vi "Fm.vi"() -> ()   [LabVIEW 2016]
uses:
  <vilib>/measure/NI_MAPro.lvlib
panel:
  out "Waveform Graph":dynamicdata(graph)
  in  "Kf":dbl(slide) scale=0.0..100.0
  in  "Fc":dbl(knob) scale=0.0..100.0
  in  "Ac":dbl(knob) scale=0.0..1.0
  in  "Am":dbl(knob) scale=0.0..1.0
  in  "Fm":dbl(knob) scale=0.0..10.0
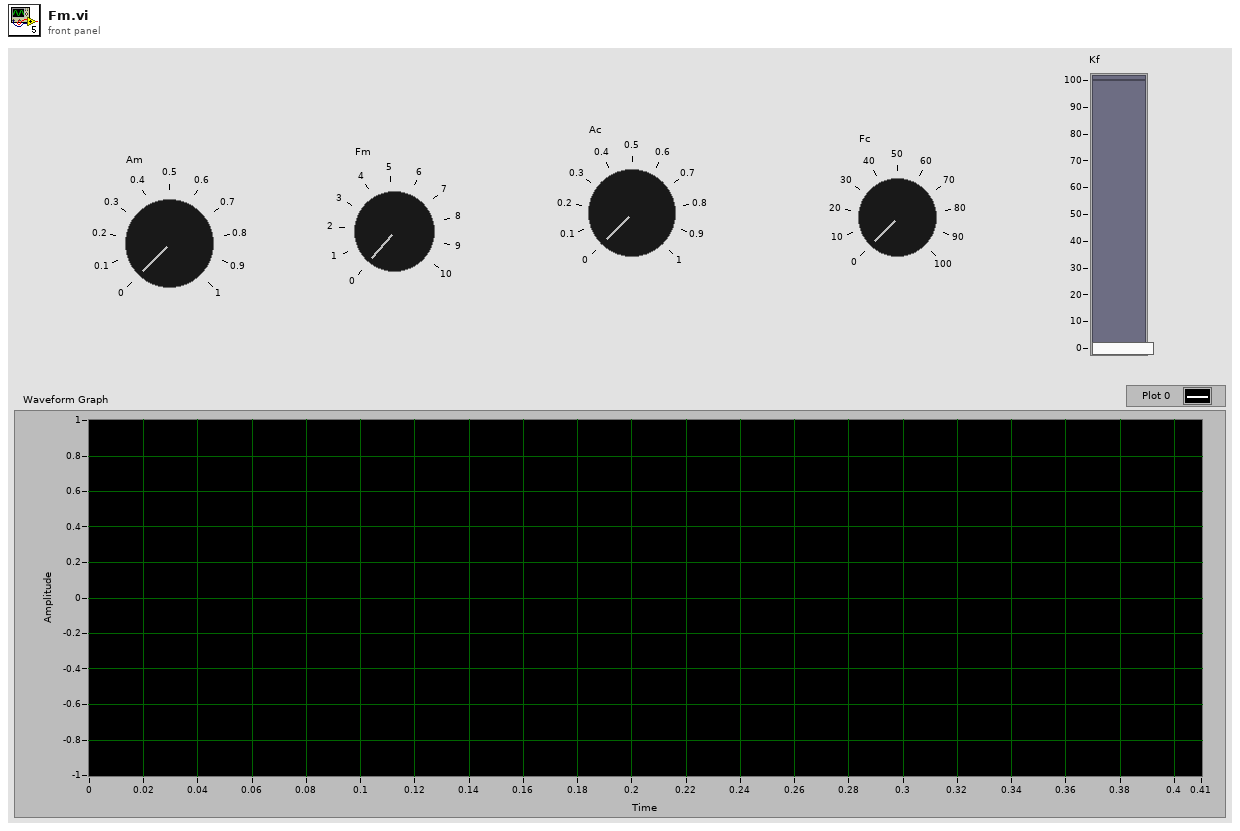
[diagram p1: front panel]
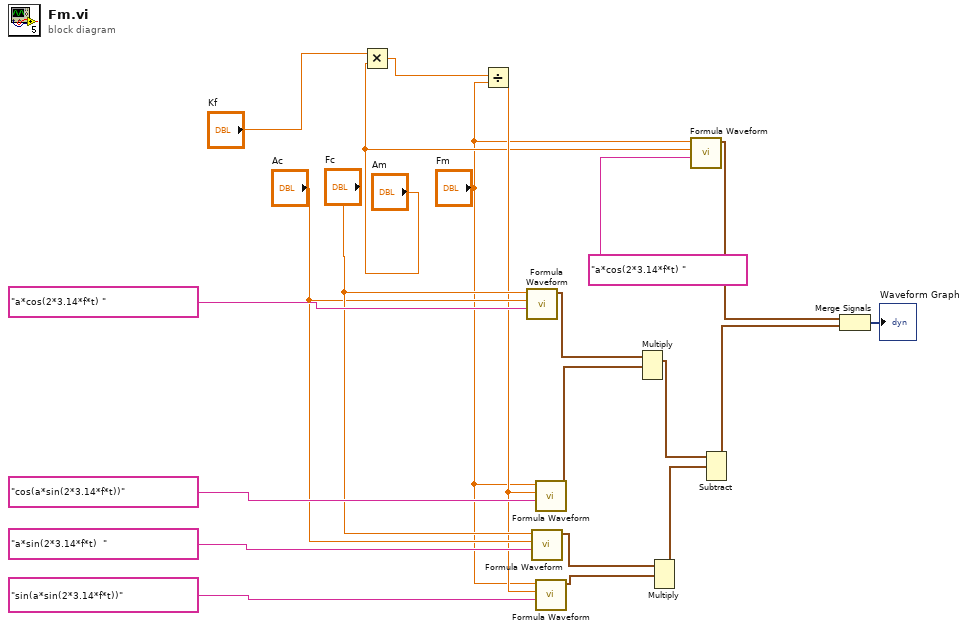
[diagram p0: block diagram]
diagram:
  n1 = Multiply(x="Kf", y="Am") -> (x*y=w14:dbl)
  n2 = Divide(x=w14, y="Fm") -> (x/y=w13:dbl)
  n3 = call <vilib>:"Formula Waveform.vi"("formula"="a*cos(2*3.14*f*t) ", "amplitude"="Ac", "frequency"="Fc") -> ("signal out"=w12:waveform(dbl))  [unwired: 7 in, 1 out]
  n4 = call <vilib>:"Formula Waveform.vi"("formula"="a*sin(2*3.14*f*t)  ", "amplitude"="Ac", "frequency"="Fc") -> ("signal out"=w10:waveform(dbl))  [unwired: 7 in, 1 out]
  n5 = call <vilib>:"Formula Waveform.vi"("formula"="cos(a*sin(2*3.14*f*t))", "amplitude"=w13, "frequency"="Fm") -> ("signal out"=w11:waveform(dbl))  [unwired: 7 in, 1 out]
  n6 = call <vilib>:"Formula Waveform.vi"("formula"="sin(a*sin(2*3.14*f*t))", "amplitude"=w13, "frequency"="Fm") -> ("signal out"=w9:waveform(dbl))  [unwired: 7 in, 1 out]
  n7 = Multiply(1:w11, 2:w12) -> (0:w8:waveform(dbl))  [unwired: 1 in, 1 out]
  n8 = Multiply(1:w9, 2:w10) -> (0:w7:waveform(dbl))  [unwired: 1 in, 1 out]
  n9 = call <vilib>:"Formula Waveform.vi"("formula"="a*cos(2*3.14*f*t) ", "amplitude"="Am", "frequency"="Fm") -> ("signal out"=w3:waveform(dbl))  [unwired: 7 in, 1 out]
  n10 = Subtract(1:w7, 2:w8) -> (0:w2:waveform(dbl))  [unwired: 1 in, 1 out]
  n11 = Merge Signals(w3, w2) -> (→"Waveform Graph":dynamicdata)
